vi "ze closure miss call.vi"(8 "error in (no error)":errorcluster, 10 "mathing_status":cluster{}, 11 "closure":cluster{}) -> (0 "error out":errorcluster)   [LabVIEW 2021, in "zenohc.lvlib"]
doc: "void ze_closure_miss_call(const struct ze_loaned_closure_miss_t *closure,\n const struct ze_miss_t *mathing_status);"
uses:
  zenohc.lvlib
  zenohc.dll
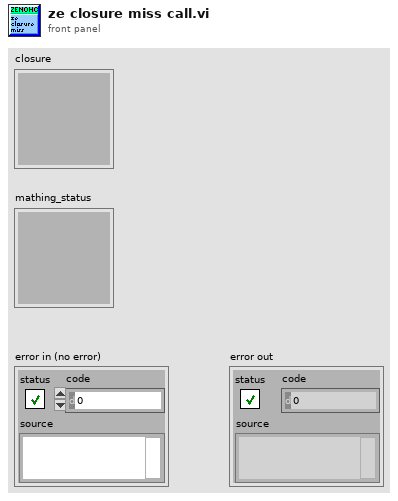
[diagram p1: front panel]
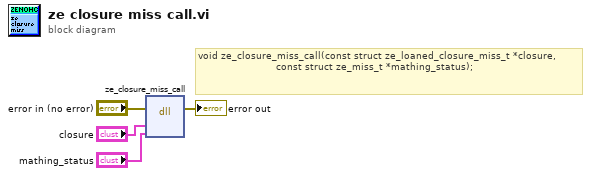
[diagram p0: block diagram]
diagram:
  # "void ze_closure_miss_call(const struct ze_loaned_closure_miss_t *closure,\n                          const struct ze_miss_t *mathing_status);"
  n1 = dll-call lib="D:/dev/zenoh_labview/zenohc/zenohc.*" fn="ze_closure_miss_call"(error in="error in (no error)", "closure"="closure", "mathing_status"="mathing_status") -> (error out=→"error out":errorcluster)  [unwired: 5 in, 1 out]
